vi "FID Manuell Kalibrieren.vi"(8 "über GT":bool, 10 "AUTO STARTEN":bool, 11 "Kalibrieren":T1) -> (2 "Wert ist im gültigen Bereich:":bool, 3 "Kalibrieren erfolgreich":bool)   [LabVIEW 2020, in "ABB-EL3000.lvlib" / "Allgemeine VI.lvlib"]
uses:
  Allgemeine VI.lvlib
  Visualisierungs Elemente/Button.ctl
  Visualisierungs Elemente/String - Ausgabefeld.ctl
  Visualisierungs Elemente/Zahlen-Ausgabefeld.ctl
  FID/FID Kalibrierung/FID Kalibrieren.ctl
  Sprachverwaltung/FGV Aktion Tabelle zerlegen.ctl
  Analysator Definition/FGV Analysator Definition Aktionen.ctl
  FGV Uras26 Aktion.ctl
  FID/FID Kalibrierung/FID Kalibrierung.lvlib
  Auto Kalibrieren/Auto Kalibrieren.lvlib
  CalGas Aufschaltung/CalGas Aufschaltung.lvlib
  Analysator Definition/Analysator Definition.lvlib
  Sprachverwaltung/Sprachverwaltung.lvlib
  Allgemein/allgemeine Sub-VIs.lvlib
panel:
  out "Rohwert CO2 high:":T2 caption="%" format="%.3f"
  out "Rohwert CO2 low:":T2 caption="ppm" format="%.3f"
  out "Rohwert O2:":T2 caption="%" format="%.3f"
  out "Raw value NMHC:":T2 caption="ppm" format="%.1f"
  in  "Kalibrierwerte kopieren?:":bool
  out "CG":T2 format="%#_5g"
  out "Titelzeile":string
  out "Raw value1 THC:":T2 caption="ppm" format="%.1f"
  out "Roh Wert THC:":T2 format="%.1f"
  out "Status":T3
  out "Einheit":T3
  out "Messbereich":T3
  out "Konzentration":T2 format="%#_5g"
  out "Name":T3
  in  "STARTEN":T4
  in  "ABBRECHEN":T4
  # "Kalibrationsgas"
  # "Konzentration"
  # "Einheit"
  # "Messbereich"
  # "ppm"
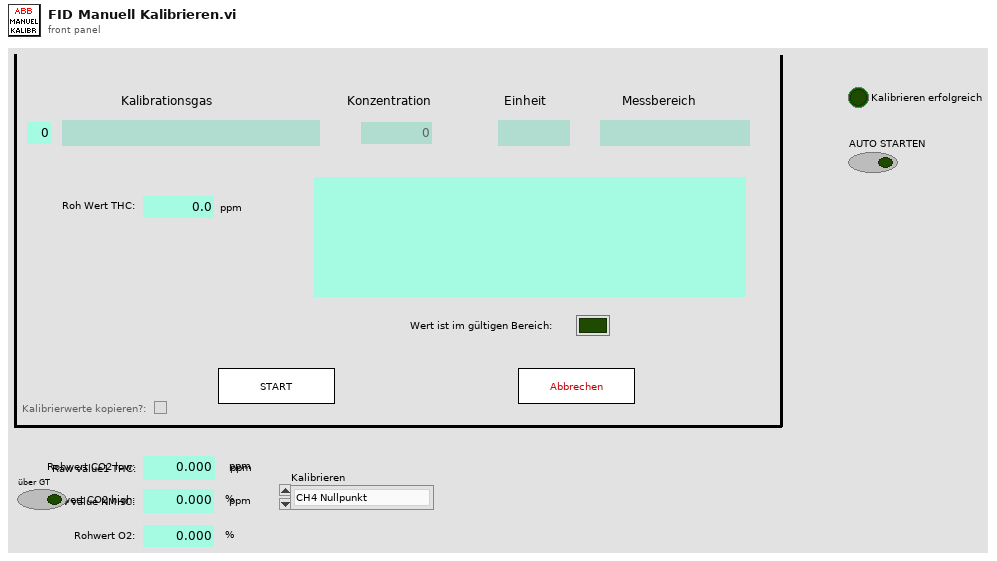
[diagram p1: front panel]
types:
  T1 = typedef "ABB-EL3000.lvlib/FID.lvlib/FID Kalibrierung.lvlib/FID Kalibrieren.ctl" = enum16{"CH4 Nullpunkt", "THC Nullpunkt", "NMHC Nullpunkt", "CH4 Endpunkt", "THC Endpunkt", "NMHC Endpunkt"}
  T2 = typedef "Zahlen-Ausgabefeld.ctl" = sgl
  T3 = typedef "String - Ausgabefeld.ctl" = string
  T4 = typedef "Button.ctl" = bool
  T5 = typedef "Sprachverwaltung.lvlib/FGV Aktion Tabelle zerlegen.ctl" = enum16{"laden", "vereinzeln", "speichern"}
  T6 = enum8{"Enabled", "Disabled", "Disabled and Grayed Out"}
  T7 = typedef "Analysator Definition.lvlib/FGV Analysator Definition Aktionen.ctl" = enum16{"lesen", "MB setzen", "MB KAL setzen", "laden"}
  T8 = typedef "Analysator Definition.lvlib/Betriebsdaten Komponente.ctl" = cluster{"Namen":string[], "MB Namen":string[], "Einheit":string, "MB Aktuell":u16, "MB Endwert":u16, "CalGase":u16[], "MB für KAL":u16[], "CG für KAL":u16[]}
  T9 = typedef "ABB-EL3000.lvlib/Allgemeine VI.lvlib/FGV Uras26 Aktion.ctl" = enum16{"lesen", "CAL-Daten laden", "Messen", "Kalibrieren vorbereiten", "Kalibrieren", "CAL-Daten speichern", "Toleranz schreiben", "CAL-Daten kopieren"}
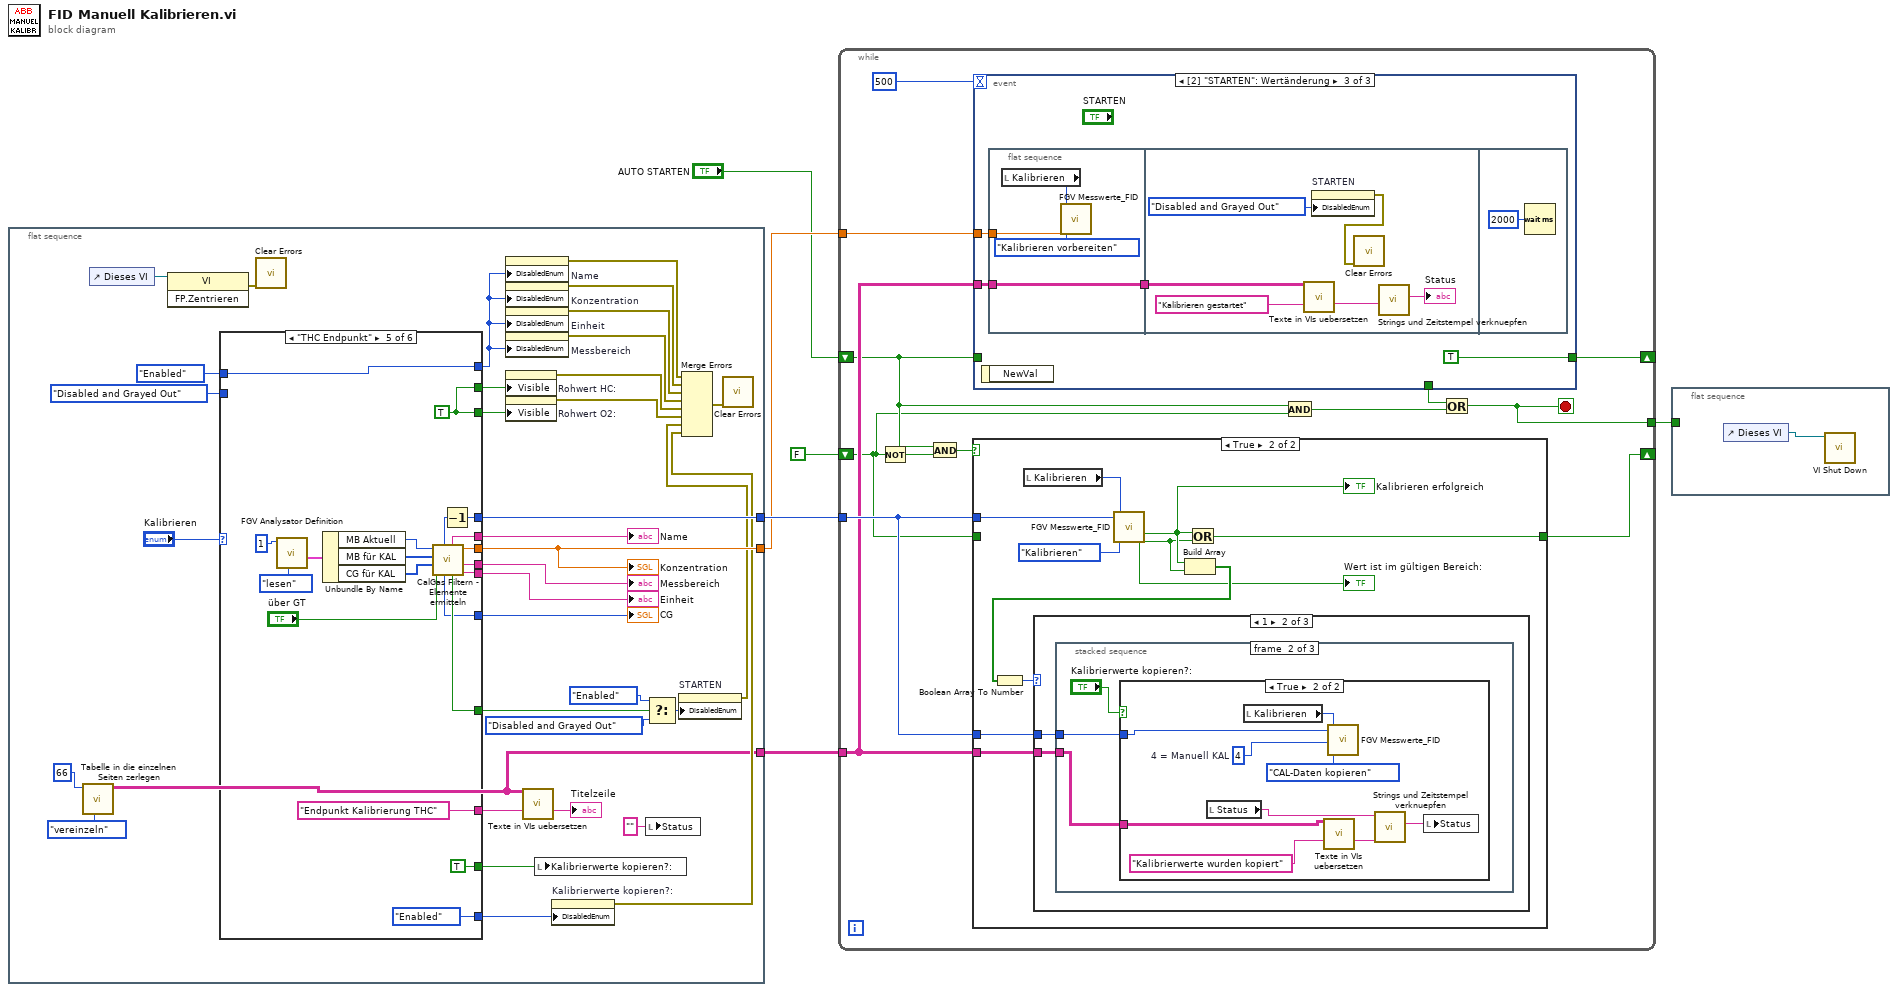
[diagram p0: block diagram]
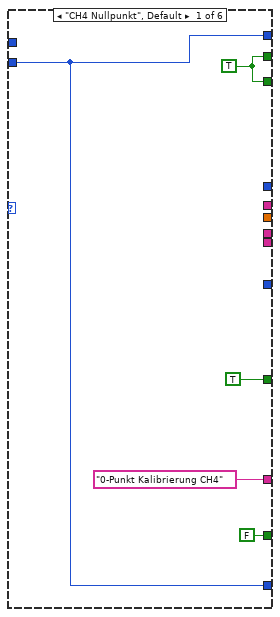
[diagram p2: hidden frame]
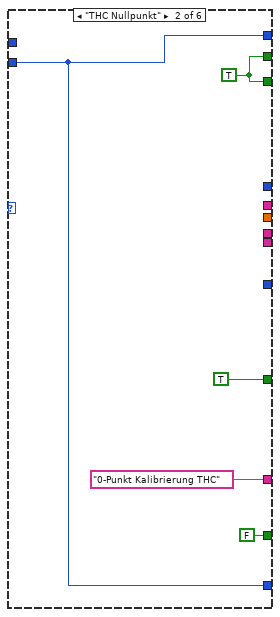
[diagram p3: hidden frame]
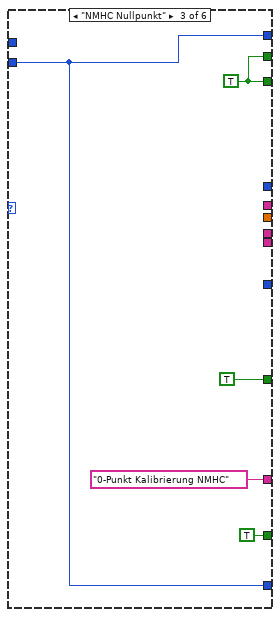
[diagram p4: hidden frame]
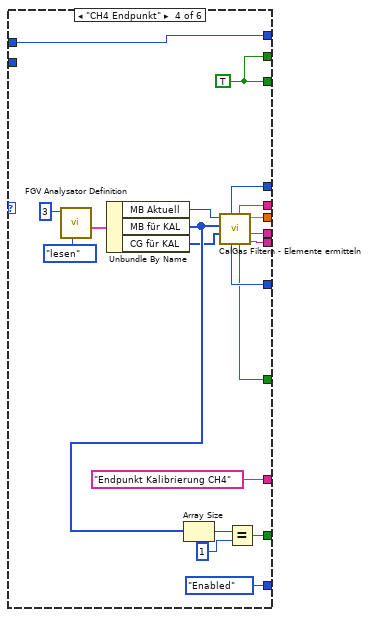
[diagram p5: hidden frame]
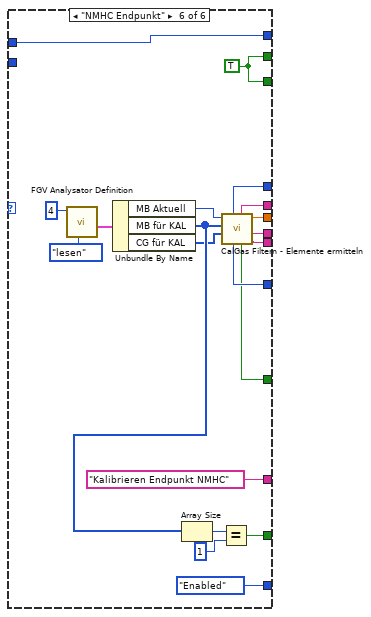
[diagram p6: hidden frame]
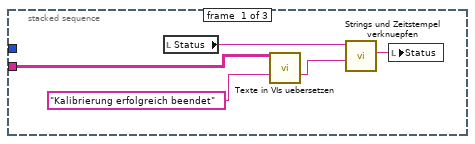
[diagram p9: hidden frame]
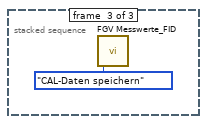
[diagram p11: hidden frame]
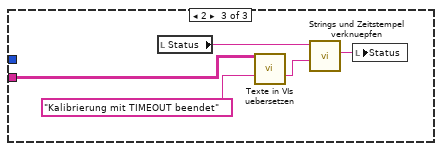
[diagram p12: hidden frame]
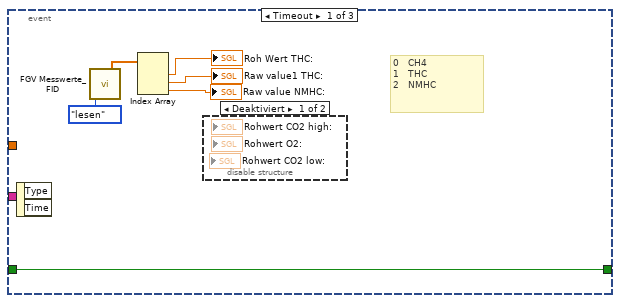
[diagram p13: hidden frame]
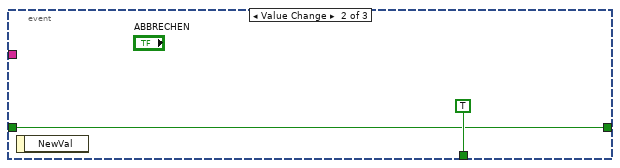
[diagram p15: hidden frame]
diagram:
  n1 = flat-sequence {
    tunnel: [w31] -> w4
    tunnel: [w35] -> w6
    tunnel: [w8] -> w2
    frame #0 {
      n2 = call "Tabelle in die einzelnen Seiten zerlegen.vi"("Aktion"=FGV_Aktion_Tabelle_zerlegen."vereinzeln", "Index (Seite)"=66) -> ("Sprachliste"=w8:string[][])  [unwired: 7 in, 2 out]
      n3 = control-ref of="Dieses VI"() -> (w13:refnum<vi>)
      n4 = invoke class="VI" method="FP.Zentrieren"(reference=w13) -> (error out=w12:errorcluster)  [unwired: 2 in, 2 out]
      n5 = case shown="\"THC Endpunkt\"" "Kalibrieren" {
        tunnel: ["0-Punkt Kalibrierung CH4" "0-Punkt Kalibrierung THC" "0-Punkt Kalibrierung NMHC" "Endpunkt Kalibrierung CH4" "Endpunkt Kalibrierung THC" "Kalibrieren Endpunkt NMHC"] -> w10
        tunnel: T6."Enabled" ("Deaktiviert") -> [_ _ _ w75 w95 w115]
        tunnel: T6."Disabled and Grayed Out" ("Deaktiviert") -> [w43 w48 w54 _ _ _]
        tunnel: [w43 w48 w54 w75 w95 w115] -> w39
        tunnel: [w42 w47 w52 w64 w86 w103] -> w37
        tunnel: [w42 w47 w52 w64 w86 w103] -> w36
        tunnel: [_ _ _ w58 w78 w113] -> w35
        tunnel: [_ _ _ w73 w92 w111] -> w31
        tunnel: [_ _ _ w74 w93 w112] -> w34
        tunnel: [_ _ _ w71 w91 w110] -> w32
        tunnel: [_ _ _ w72 w90 w114] -> w33
        tunnel: [TRUE TRUE TRUE w69 w89 w108] -> w30
        tunnel: [_ _ _ w70 w88 w109] -> w28
        tunnel: [FALSE FALSE TRUE w65 TRUE w105] -> w25
        tunnel: [w43 w48 w54 T6."Enabled" ("Deaktiviert") T6."Enabled" ("Deaktiviert") T6."Enabled" ("Deaktiviert")] -> w24
        frame "CH4 Nullpunkt", Default {
          w42 = TRUE
        }
        frame "THC Nullpunkt" {
          w47 = TRUE
        }
        frame "NMHC Nullpunkt" {
          w52 = TRUE
        }
        frame "CH4 Endpunkt" {
          w64 = TRUE
          n6 = call "FGV Analysator Definition.vi"("Aktionen"=FGV_Analysator_Definition_Aktionen."lesen", "Komponente"=3) -> ("Betriebsdaten Komponente"=w63:T8)  [unwired: 5 in, 4 out]
          n7 = Unbundle By Name(w63) -> ("MB Aktuell"=w57:u16, "MB für KAL"=w60:u16[], "CG für KAL"=w59:u16[])
          n8 = Array Size(array=w60) -> (size(s)=w67:i32)
          n9 = call "CalGas Filtern - Elemente ermitteln.vi"("CalGase"=w59, "MB KAL"=w60, "derzeitiger Messbereich"=w57) -> ("Einheit"=w72:T3, "Messberich"=w71:T3, "Wert 1"=w73:T2, "OK"=w69:bool, "Name"=w74:T3, "CalGas"=w70:i32, "Messbereich"=w58:u16)  [unwired: 1 in, 1 out]
          n10 = Equal?(x=w67, y=1) -> (x = y?=w65:bool)
        }
        frame "THC Endpunkt" {
          w86 = TRUE
          n11 = call "FGV Analysator Definition.vi"("Aktionen"=FGV_Analysator_Definition_Aktionen."lesen", "Komponente"=1) -> ("Betriebsdaten Komponente"=w84:T8)  [unwired: 5 in, 4 out]
          n12 = Unbundle By Name(w84) -> ("MB Aktuell"=w81:u16, "MB für KAL"=w80:u16[], "CG für KAL"=w79:u16[])
          n13 = call "CalGas Filtern - Elemente ermitteln.vi"("über GT"="über GT", "CalGase"=w79, "MB KAL"=w80, "derzeitiger Messbereich"=w81) -> ("Einheit"=w90:T3, "Messberich"=w91:T3, "Wert 1"=w92:T2, "OK"=w89:bool, "Name"=w93:T3, "CalGas"=w88:i32, "Messbereich"=w94:u16)  [unwired: 1 out]
          n14 = Decrement(x=w94) -> (x-1=w78:u16)
        }
        frame "NMHC Endpunkt" {
          w103 = TRUE
          n15 = call "FGV Analysator Definition.vi"("Aktionen"=FGV_Analysator_Definition_Aktionen."lesen", "Komponente"=4) -> ("Betriebsdaten Komponente"=w102:T8)  [unwired: 5 in, 4 out]
          n16 = Unbundle By Name(w102) -> ("MB Aktuell"=w99:u16, "MB für KAL"=w98:u16[], "CG für KAL"=w97:u16[])
          n17 = Array Size(array=w98) -> (size(s)=w107:i32)
          n18 = Equal?(x=w107, y=1) -> (x = y?=w105:bool)
          n19 = call "CalGas Filtern - Elemente ermitteln.vi"("CalGase"=w97, "MB KAL"=w98, "derzeitiger Messbereich"=w99) -> ("Einheit"=w114:T3, "Messberich"=w110:T3, "Wert 1"=w111:T2, "OK"=w108:bool, "Name"=w112:T3, "CalGas"=w109:i32, "Messbereich"=w113:u16)  [unwired: 1 in, 1 out]
        }
      }
      "Name" <- w34
      "Konzentration" <- w31
      "Messbereich" <- w32
      "Einheit" <- w33
      "CG" <- w28
      n20 = call <vilib>:"Clear Errors.vi"("error in (no error)"=w12) -> ()  [unwired: 5 in, 2 out]
      n21 = property on="Name" class="Str (strikt)"("DisabledEnum"=w39) -> (error out=w23:errorcluster)  [unwired: 2 in, 1 out]
      n22 = property on="Konzentration" class="DigWert (strikt)"("DisabledEnum"=w39) -> (error out=w22:errorcluster)  [unwired: 2 in, 1 out]
      n23 = property on="Einheit" class="Str (strikt)"("DisabledEnum"=w39) -> (error out=w21:errorcluster)  [unwired: 2 in, 1 out]
      n24 = property on="Messbereich" class="Str (strikt)"("DisabledEnum"=w39) -> (error out=w20:errorcluster)  [unwired: 2 in, 1 out]
      n25 = property on="Rohwert HC:" class="DigWert (strikt)"("Visible"=w37) -> (error out=w19:errorcluster)  [unwired: 2 in, 1 out]
      n26 = property on="Rohwert O2:" class="DigWert (strikt)"("Visible"=w36) -> (error out=w18:errorcluster)  [unwired: 2 in, 1 out]
      n27 = call "Texte in VIs uebersetzen.vi"("Sprachliste"=w8, "String zum Übersetzen"=w10) -> ("String zum Übersetzen"=→"Titelzeile":string)  [unwired: 9 in, 4 out]
      n28 = local write "Kalibrierwerte kopieren?:"(w25) -> ()
      n29 = property on="Kalibrierwerte kopieren?:" class="Bool. (strikt)"("DisabledEnum"=w24) -> (error out=w15:errorcluster)  [unwired: 2 in, 1 out]
      n30 = local write "Status"(T3 "" ("Status")) -> ()
      n31 = Select(t=T6."Enabled" ("Deaktiviert"), s=w30, f=T6."Disabled and Grayed Out" ("Deaktiviert")) -> (s? t:f=w29:T6)
      n32 = property on="STARTEN" class="Bool."("DisabledEnum"=w29) -> (error out=w16:errorcluster)  [unwired: 2 in, 1 out]
      n33 = Merge Errors(w23, w22, w21, w20, w19, w18, w16, w15) -> (w17:errorcluster)
      n34 = call <vilib>:"Clear Errors.vi"("error in (no error)"=w17) -> ()  [unwired: 5 in, 2 out]
    }
  }
  n35 = while {
    shift-right: [w128] -> _
    shift-left: "AUTO STARTEN" -> [w119]
    tunnel: w6 -> [w122]
    shift-right: [w127] -> _
    shift-left: FALSE ("STARTEN") -> [w117]
    tunnel: w4 -> [w124]
    tunnel: [w120] -> w3
    tunnel: w2 -> [w121]
    stop <- w120 stop-if-true
    n36 = Not(x=w117) -> (.not. x?=w126:bool)
    n37 = And(x=w119, y=w126) -> (x .and. y?=w125:bool)
    n38 = case shown="True" w125 {
      tunnel: w122 -> [_ w136]
      tunnel: [w130 w141] -> w127
      tunnel: w117 -> [w130 _]
      tunnel: w122 -> [_ w135]
      tunnel: w121 -> [_ w131]
      frame False {
      }
      frame True {
        n39 = local read "Kalibrieren"() -> (w133:T1)
        n40 = call "FGV Messwerte_FID.vi"("Messbereich"=w136, "Kalibrieren"=w133, "Aktion"=FGV_Uras26_Aktion."Kalibrieren") -> ("im gültigen Bereich"=→"Wert ist im gültigen Bereich:":bool, "Kalibrieren erfolgreich"=w140:bool, "CAL TimeOut"=w139:bool)  [unwired: 17 in, 5 out]
        "Kalibrieren erfolgreich" <- w140
        n41 = Build Array(w140, w139) -> (w138:bool[])
        n42 = Boolean Array To Number(Boolean array=w138) -> (number=w137:u32)
        n43 = case shown="1" w137 {
          tunnel: w135 -> [_ w143 _]
          tunnel: w131 -> [_ w142 w163]
          frame 0, Default {
          }
          frame 1 {
            n44 = stacked-sequence {
              tunnel: w143 -> [_ w151 _]
              tunnel: w142 -> [w146 w149 _]
              frame #0 {
                n45 = local read "Status"() -> (w147:T3)
                n46 = call "Texte in VIs uebersetzen.vi"("Sprachliste"=w146, "String zum Übersetzen"="Kalibrierung erfolgreich beendet" ("String 1 hinzufügen")) -> ("String zum Übersetzen"=w144:string)  [unwired: 9 in, 4 out]
                n47 = call "Strings und Zeitstempel verknuepfen.vi"("String 1 hinzufügen"=w144, "Eingagns String"=w147) -> ("Verknüpfter String"=w148:string)  [unwired: 9 in]
                n48 = local write "Status"(w148) -> ()
              }
              frame #1 {
                n49 = case shown="True" "Kalibrierwerte kopieren?:" {
                  tunnel: w151 -> [_ w152]
                  tunnel: w149 -> [_ w154]
                  frame False {
                  }
                  frame True {
                    w153 = u16 4  # 4 = Manuell KAL
                    n50 = local read "Status"() -> (w159:T3)
                    n51 = local read "Kalibrieren"() -> (w157:T1)
                    n52 = call "Texte in VIs uebersetzen.vi"("Sprachliste"=w154, "String zum Übersetzen"="Kalibrierwerte wurden kopiert" ("String 1 hinzufügen")) -> ("String zum Übersetzen"=w156:string)  [unwired: 9 in, 4 out]
                    n53 = call "FGV Messwerte_FID.vi"("Messbereich"=w152, "Zielmessbereich"=w153, "Kalibrieren"=w157, "Aktion"=FGV_Uras26_Aktion."CAL-Daten kopieren") -> ()  [unwired: 16 in, 8 out]
                    n54 = call "Strings und Zeitstempel verknuepfen.vi"("String 2 hinzufügen"=w156, "Eingagns String"=w159) -> ("Verknüpfter String"=w160:string)  [unwired: 9 in]
                    n55 = local write "Status"(w160) -> ()
                  }
                }
              }
              frame #2 {
                n56 = call "FGV Messwerte_FID.vi"("Aktion"=FGV_Uras26_Aktion."CAL-Daten speichern") -> ()  [unwired: 19 in, 8 out]
              }
            }
          }
          frame 2 {
            n57 = local read "Status"() -> (w166:T3)
            n58 = call "Texte in VIs uebersetzen.vi"("Sprachliste"=w163, "String zum Übersetzen"="Kalibrierung mit TIMEOUT beendet" ("String 1 hinzufügen")) -> ("String zum Übersetzen"=w162:string)  [unwired: 9 in, 4 out]
            n59 = call "Strings und Zeitstempel verknuepfen.vi"("String 1 hinzufügen"=w162, "Eingagns String"=w166) -> ("Verknüpfter String"=w165:string)  [unwired: 9 in]
            n60 = local write "Status"(w165) -> ()
          }
        }
        n61 = Or(x=w140, y=w139) -> (x .or. y?=w141:bool)
      }
    }
    n62 = event shown="[2] \"STARTEN\": Wertänderung" {
      selector: _ -> [_ _ _]
      dyn-events: _ -> [_ _ _]
      timeout: 500 -> [_ _ _]
      tunnel: [_ TRUE ("ABBRECHEN") _] -> w123
      tunnel: [w172 w173 TRUE ("STARTEN")] -> w128
      tunnel: w119 -> [w172 w173 _]
      tunnel: w124 -> [_ _ w177]
      tunnel: w121 -> [_ _ w175]
      event Timeout {
        # "0   CH4\n1   THC\n2   NMHC"
        n63 = event-data() -> ()  [unwired: 1 in, 2 out]
        n64 = call "FGV Messwerte_FID.vi"("Aktion"=FGV_Uras26_Aktion."lesen") -> ("Rohwerte"=w170:sgl[])  [unwired: 19 in, 7 out]
        n65 = Index Array(array=w170) -> (element #1=→"Roh Wert THC:":sgl, element #2=→"Raw value1 THC:":sgl, element #3=→"Raw value NMHC:":sgl)  [unwired: 3 in]
        n66 = disable-structure shown="Deaktiviert" {
          frame Disabled {
          }
          frame Enabled {
          }
        }
      }
      event Value Change {
        n67 = event-data() -> ()  [unwired: 1 in, 1 out]
      }
      event Value Change {
        n68 = event-data() -> ()  [unwired: 1 in, 1 out]
        n69 = flat-sequence {
          tunnel: w177 -> [w181]
          tunnel: w175 -> [w179]
          tunnel: [w179] -> w176
          tunnel: w176 -> [w183]
          frame #0 {
            n70 = local read "Kalibrieren"() -> (w180:T1)
            n71 = call "FGV Messwerte_FID.vi"("Prüfgaskonz."=w181, "Kalibrieren"=w180, "Aktion"=FGV_Uras26_Aktion."Kalibrieren vorbereiten") -> ()  [unwired: 17 in, 8 out]
          }
          frame #1 {
            n72 = call "Texte in VIs uebersetzen.vi"("Sprachliste"=w183, "String zum Übersetzen"="Kalibrieren gestartet" ("String 1 hinzufügen")) -> ("String zum Übersetzen"=w184:string)  [unwired: 9 in, 4 out]
            n73 = property on="STARTEN" class="Bool."("DisabledEnum"=T6."Disabled and Grayed Out" ("Deaktiviert")) -> (error out=w186:errorcluster)  [unwired: 2 in, 1 out]
            n74 = call <vilib>:"Clear Errors.vi"("error in (no error)"=w186) -> ()  [unwired: 5 in, 2 out]
            n75 = call "Strings und Zeitstempel verknuepfen.vi"("String 1 hinzufügen"=w184) -> ("Verknüpfter String"=→"Status":string)  [unwired: 10 in]
          }
          frame #2 {
            n76 = Wait (ms)(milliseconds to wait=u32 2000 ("Zu wartende ms")) -> ()  [unwired: 1 out]
          }
        }
      }
    }
    n77 = And(x=w119, y=w117) -> (x .and. y?=w118:bool)
    n78 = Or(x=w123, y=w118) -> (x .or. y?=w120:bool)
  }
  n79 = flat-sequence {
    tunnel: w3 -> [_]
    frame #0 {
      n80 = control-ref of="Dieses VI"() -> (w190:refnum<vi>)
      n81 = call "VI Shut Down.vi"("VI Referenz"=w190) -> ()  [unwired: 11 in]
    }
  }
